vi "x1e-6(SubVI).vi"(1 "in":dbl) -> (0 "out":dbl)   [LabVIEW 2024]
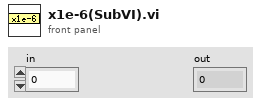
[diagram p1: front panel]
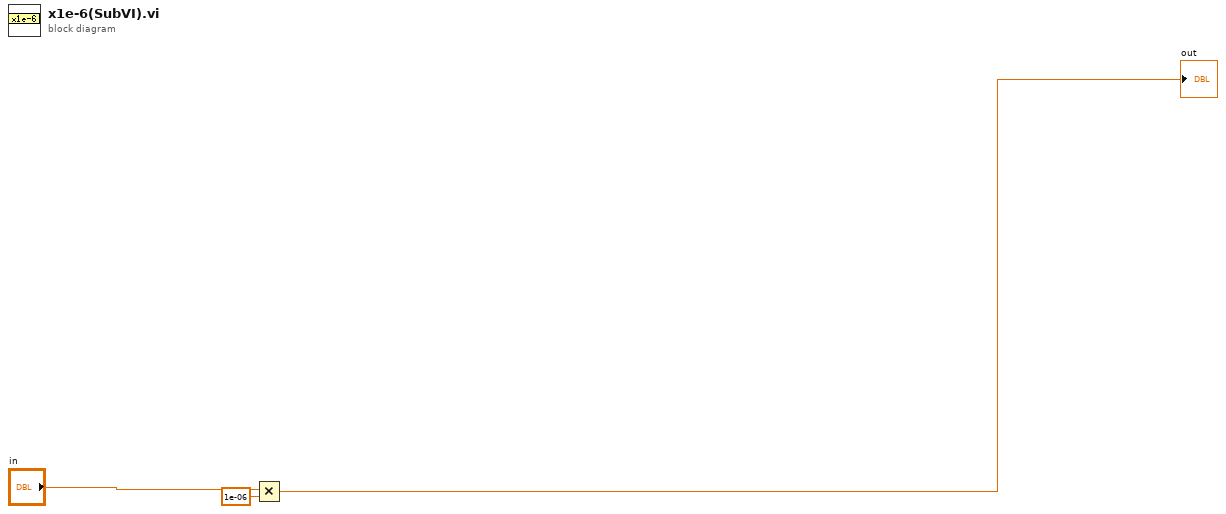
[diagram p0: block diagram]
diagram:
  n1 = Multiply(x="in", y=1e-06 ("x")) -> (x*y=→"out":dbl)
